vi "MMC_getPos.vi"(3 "Error in":errorcluster) -> (0 "Error out":errorcluster, 2 "current position":i32)   [LabVIEW 2024]
doc: "This vi reads the current motor position"
uses:
  MMC.dll
panel:
  # "MMC_getPos"
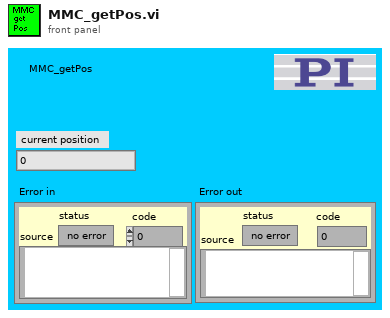
[diagram p1: front panel]
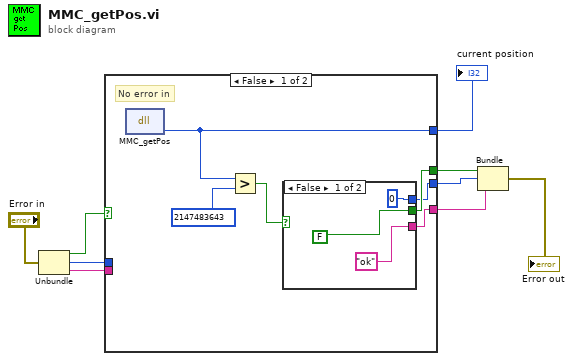
[diagram p0: block diagram]
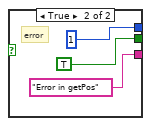
[diagram p2: hidden frame]
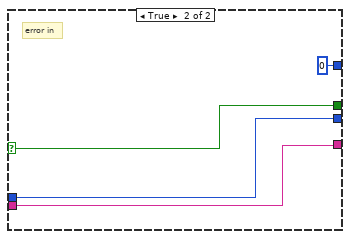
[diagram p3: hidden frame]
diagram:
  n1 = Unbundle("Error in") -> ("status"=w4:bool, "code"=w2:i32, "source"=w3:string)
  n2 = case shown="False" w4 {
    selector: w4 -> [_ w23]
    tunnel: [w10 w24] -> w9
    tunnel: [w11 w23] -> w8
    tunnel: [w12 w25] -> w6
    tunnel: w3 -> [_ w25]
    tunnel: w2 -> [_ w24]
    tunnel: [w14 0] -> w1
    frame False {
      # "No error in"
      n3 = dll-call lib="E:/Wilson/HoppingSICM_TK/HoppingSICM_v1/DLLs/MMC.dll" fn="MMC_getPos"() -> (w14:i32)  [unwired: 3 in, 2 out]
      n4 = Greater?(x=w14, y=2147483643) -> (0:w15:bool)
      n5 = case shown="False" w15 {
        tunnel: ["ok" "Error in getPos"] -> w12
        tunnel: [FALSE TRUE] -> w11
        tunnel: [0 1] -> w10
        frame False {
        }
        frame True {
          # "error"
        }
      }
    }
    frame True {
      # "error in"
    }
  }
  "current position" <- w1
  n6 = Bundle(w8, "code"=w9, "source"=w6) -> (→"Error out":cluster{bool, "code":i32, "source":string})  [unwired: 1 in]
